vi "tcp_client.vi"() -> ()   [LabVIEW 2019]
panel:
  in  "interval":u32=2000
  in  "timeout":i32=100
  in  "port":u16=10000
  in  "addr":string="192.168.24.181"
  out "status":bool
  out "client_step":i32
  in  "stop":bool
  out "value":dbl[](array[numeric]) format="%_6f"
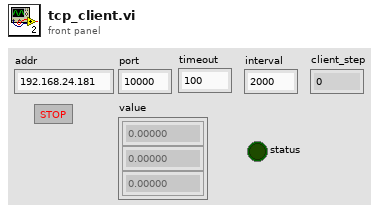
[diagram p1: front panel]
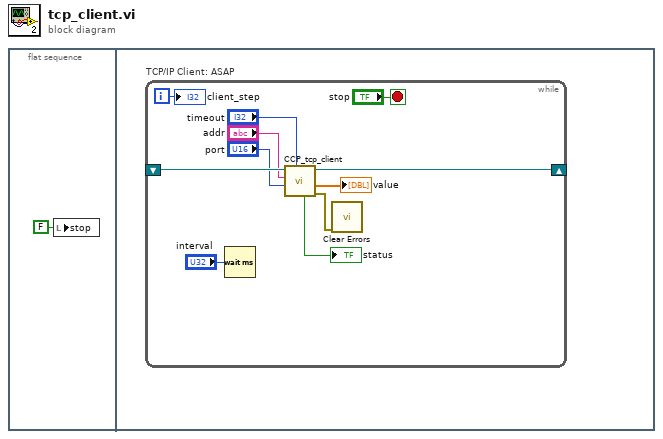
[diagram p0: block diagram]
diagram:
  n1 = flat-sequence {
    frame #0 {
      n2 = local write "stop"(FALSE ("stop")) -> ()
    }
    frame #1 {
      n3 = while "TCP/IP Client: ASAP" {
        shift-right: [w8] -> _
        shift-left: _ -> [w9]
        i -> [w10]
        stop <- "stop" stop-if-true
        n4 = Wait (ms)(milliseconds to wait="interval") -> ()  [unwired: 1 out]
        n5 = call "CCP_tcp_client.vi"("wait_time"="timeout", "port"="port", "address"="addr", "conn_id_in"=w9) -> ("error out"=w3:errorcluster, "array_value"=→"value":dbl[], "conn_id_out"=w8:refnum<k5>, "status"=→"status":bool)  [unwired: 3 in, 1 out]
        n6 = call <vilib>:"Clear Errors.vi"("error in (no error)"=w3) -> ()  [unwired: 5 in, 2 out]
        "client_step" <- w10
      }
    }
  }
